vi "Write View Settings.vi"(0 "Controller Actor in":refnum<class "Controller Actor.lvclass">, 1 "View Name":string, 3 "View Settings":T1, 5 "error in (no error)":errorcluster) -> (14 "Controller Actor out":refnum<class "Controller Actor.lvclass">, 19 "error out":errorcluster)   [LabVIEW 2016, in "Event Actors.lvlib" / "Controller Actor.lvclass"]
doc: "Allows to set the View behavior by setting the following flags:\n\n<b>Exclude From Broadcast</b>: message originating form another sink will not be broadcasted to the sink being cosidered\n<b>Paused</b>: the sink will not send events and will not receive them anymore\n<b>Receive only</b>: The sing will receive events but not send any"
uses:
  Controller Actor.lvclass
  View Settings.ctl
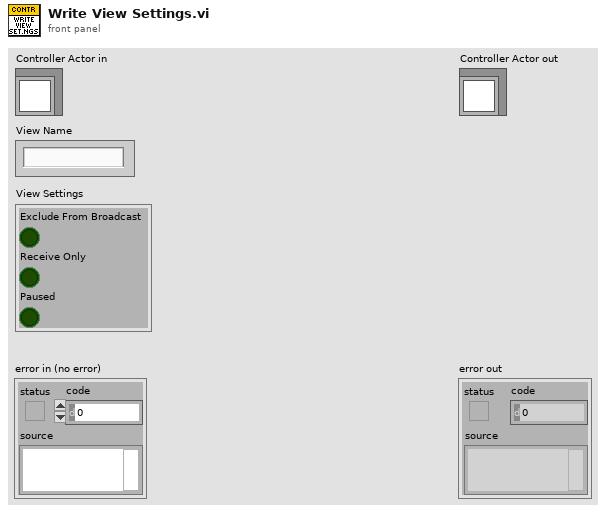
[diagram p1: front panel]
types:
  T1 = typedef "Event Actors.lvlib/Controller Actor.lvclass/View Settings.ctl" = cluster{"Exclude From Broadcast":bool, "Receive Only":bool, "Paused":bool}
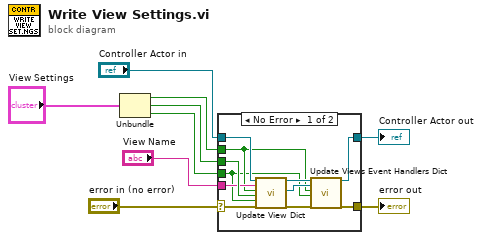
[diagram p0: block diagram]
diagram:
  n1 = Unbundle("View Settings") -> ("Exclude From Broadcast"=w3:bool, "Receive Only"=w1:bool, "Paused"=w2:bool)
  n2 = case shown="No Error" "error in (no error)" {
    selector: "error in (no error)" -> [w20 w22]
    tunnel: [w15 w22] -> w8
    tunnel: [w13 w21] -> w6
    tunnel: "Controller Actor in" -> [w19 w21]
    tunnel: "View Name" -> [w17 _]
    tunnel: w3 -> [w11 _]
    tunnel: w1 -> [w18 _]
    tunnel: w2 -> [w10 _]
    frame No Error {
      n3 = call "Update View Dict.vi"("Controller Actor in"=w19, "View Name"=w17, "Exclude From Broadcast (F)"=w11, "Receive Only (F)"=w18, "Paused (F)"=w10, "error in (no error)"=w20) -> ("Controller Actor out"=w14:refnum<class "Controller Actor.lvclass">, "View Enququer"=w12:refnum<class "Message Enqueuer.lvclass">, "error out"=w16:errorcluster)  [unwired: 11 in]
      n4 = call "Update Views Event Handlers Dict.vi"("Controller Actor in"=w14, "View Enququer"=w12, "Exclude From Broadcast (F)"=w11, "Paused (F)"=w10, "error in (no error)"=w16) -> ("Controller Actor out"=w13:refnum<class "Controller Actor.lvclass">, "error out"=w15:errorcluster)  [unwired: 13 in]
    }
    frame Error {
    }
  }
  "error out" <- w8
  "Controller Actor out" <- w6
